vi "Configure Channels.vi"(8 "error in":errorcluster, 11 "AI Voltage DAQmx Cont CFG in":refnum<class "AI Voltage DAQmx Cont CFG.lvclass">) -> (0 "error out":errorcluster, 3 "AI Voltage DAQmx Cont CFG out":refnum<class "AI Voltage DAQmx Cont CFG.lvclass">)   [LabVIEW 2024, in "AI Voltage DAQmx Cont CFG.lvclass"]
uses:
  AI Voltage DAQmx Cont CFG.lvclass
  DAQmx BufferLastReadsDBL/DAQmx BufferLastReadsDBL.lvclass/DAQmx BufferLastReadsDBL.ctl
  DAQmx Base CFG/DAQmx Base CFG.lvclass/DAQmx Base CFG.ctl
  Configurations/CFG Base/CFG Base.lvclass/CFG Base.ctl
  a8fa0662-019b-449f-adcc-c346202d0b6d.vi
  a8fa0662-019b-449f-adcc-c346202d0b6d.vi/a4169a97-72fc-4003-a778-603cf20cafa0.vi
  <vilib>/JDP Science/JSONtext/Find Item.vi
  <vilib>/JDP Science/JSONtext/Next JSON Value.vi
  <vilib>/JDP Science/JSONtext/String Subset.vi
  <vilib>/JDP Science/JSONtext/Parsing/Advance past next JSON Value (inlined COPY).vi
  <vilib>/JDP Science/JSONtext/Parsing/Advance past whitespace.vi
  <vilib>/JDP Science/JSONtext/Parsing/Advance past String.vi
  <vilib>/JDP Science/JSONtext/Parsing/Advance past Number.vi
  <vilib>/JDP Science/JSONtext/Parsing/Advance past Line Ending.vi
  <vilib>/JDP Science/JSONtext/Parsing/Parse Full Path or Item Name.vi
  <vilib>/JDP Science/JSONtext/Parsing/Advance past Array.vi
  <vilib>/JDP Science/JSONtext/Parsing/Advance past Object.vi
  <vilib>/JDP Science/JSONtext/support/Error Cluster From Code.vi
  <vilib>/JDP Science/JSONtext/Offset/Find Item Locations by Path.vi
  <vilib>/JDP Science/JSONtext/JSON text to Variant.vi
  <vilib>/Utility/error.llb/Error Cluster From Error Code.vi
  <vilib>/DAQmx/create/channels.llb/DAQmx Create Channel (AI-Voltage-Basic).vi
  <vilib>/JDP Science/JSONtext/LVClass Serializer/JSONtext LVClass Serializer.lvclass
  DAQmx Base CFG/DAQmx Base CFG.lvclass
  DAQmx BufferLastReadsDBL/DAQmx BufferLastReadsDBL.lvclass
  Buffers/BufferLastReadingsDBL/BufferLastReadsDBL.lvclass
  Configurations/CFG Base/CFG Base.lvclass
  Configurations/CFG JSON/CFG JSON.lvclass
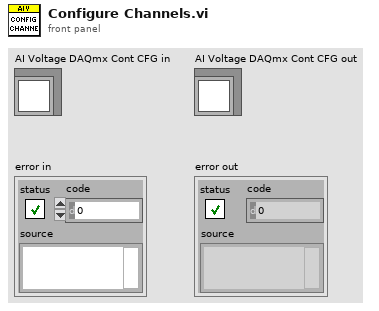
[diagram p1: front panel]
types:
  T1 = cluster{"Name":string, "Enabled":bool, "Max Value":dbl, "Min Value":dbl, "Input Terminal CFG":string, "Units":string}[]
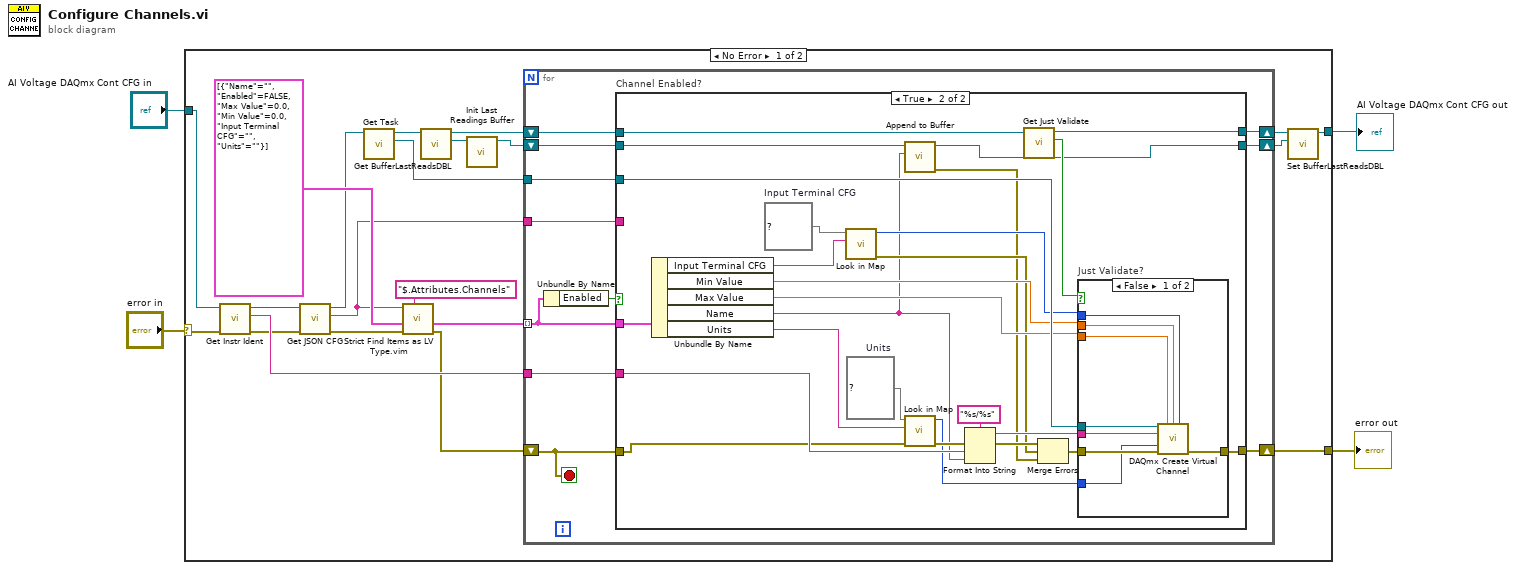
[diagram p0: block diagram]
diagram:
  n1 = case shown="No Error" "error in" {
    selector: "error in" -> [w19 w74]
    tunnel: "AI Voltage DAQmx Cont CFG in" -> [w16 w75]
    tunnel: [w20 w74] -> w1
    tunnel: [w6 w75] -> w2
    frame No Error {
      n2 = call-dynamic "Get Instr Ident.vi"("error in"=w19, "CFG JSON in"=w16) -> ("error out"=w14:errorcluster, "Instr Ident"=w21:string, "CFG JSON out"=w22:refnum<class "AI Voltage DAQmx Cont CFG.lvclass">)  [unwired: 7 in]
      n3 = call "Get JSON CFG.vi"("CFG JSON in"=w22) -> ("<JSON> CFG"=w18:string, "CFG JSON out"=w13:refnum<class "AI Voltage DAQmx Cont CFG.lvclass">)  [unwired: 9 in]
      n4 = call "Get Task.vi"("DAQmx Base CFG in"=w13) -> ("Task"=w12:refnum<k21>, "DAQmx Base CFG out"=w10:refnum<class "AI Voltage DAQmx Cont CFG.lvclass">)  [unwired: 9 in]
      n5 = call "Strict Find Items as LV Type.vim"("$Path or Item Name"="$.Attributes.Channels", "error in"=w14, "Data Type and Default Value"=T1 [{"Name"="", "Enabled"=FALSE, "Max Value"=0.0, "Min Value"=0.0, "Input Terminal CFG"="", "Units"=""}], "<JSON>"=w18) -> ("error out"=w7:errorcluster, "Data out"=w17:T1)  [unwired: 5 in, 1 out]
      n6 = call "Get BufferLastReadsDBL.vi"("DAQmx BufferLastReadsDBL in"=w10) -> ("BufferLastReadsDBL.lvclass"=w8:refnum<class "BufferLastReadsDBL.lvclass">, "DAQmx BufferLastReadsDBL out"=w9:refnum<class "AI Voltage DAQmx Cont CFG.lvclass">)  [unwired: 9 in]
      n7 = call "Init Last Readings Buffer.vi"("BufferLastReadingsDBL in"=w8) -> ("BufferLastReadingsDBL out"=w11:refnum<class "BufferLastReadsDBL.lvclass">)  [unwired: 9 in, 1 out]
      n8 = for {
        tunnel: w17 -> [w32] mode=indexing
        shift-right: [w35] -> w20
        shift-left: w7 -> [w34]
        tunnel: w21 -> [w33]
        tunnel: w18 -> [w31]
        tunnel: w12 -> [w30]
        shift-right: [w29] -> w15
        shift-left: w9 -> [w28]
        shift-right: [w25] -> w5
        shift-left: w11 -> [w26]
        stop <- w34 stop-if-true
        n9 = Unbundle By Name(w32) -> ("Enabled"=w27:bool)
        n10 = case "Channel Enabled?" shown="True" w27 {
          tunnel: [w38 w63] -> w35
          tunnel: w34 -> [w38 w45]
          tunnel: w33 -> [_ w57]
          tunnel: w32 -> [_ w64]
          tunnel: [w37 w60] -> w29
          tunnel: w31 -> [_ _]
          tunnel: w30 -> [_ w62]
          tunnel: w28 -> [w37 w61]
          tunnel: w26 -> [w36 w44]
          tunnel: [w36 w39] -> w25
          frame False {
          }
          frame True {
            w40 = map{string, i32} {"Default"=-1, "Differential"=10106, "NRSE"=10078, "Pseudodifferential"=12529, "RSE"=10083}  # Input Terminal CFG
            w41 = map{string, i32} {"From Custom Scale"=10065, "Volts"=10348}  # Units
            n11 = Unbundle By Name(w64) -> ("Input Terminal CFG"=w53:string, "Min Value"=w51:dbl, "Max Value"=w50:dbl, "Name"=w43:string, "Units"=w48:string)
            n12 = call "Look in Map.vi"("Key"=w53, "Map"=w40) -> ("error out"=w47:errorcluster, "Value"=w52:i32)  [unwired: 8 in]
            n13 = call "Append to Buffer.vi"("Channel"=w43, "BufferLastReadingsDBL in"=w44) -> ("error out"=w42:errorcluster, "BufferLastReadingsDBL out"=w39:refnum<class "BufferLastReadsDBL.lvclass">)  [unwired: 8 in]
            n14 = call "Look in Map.vi"("error in"=w45, "Key"=w48, "Map"=w41) -> ("error out"=w49:errorcluster, "Value"=w46:i32)  [unwired: 7 in]
            n15 = Format Into String(format string="%s/%s", error in=w49, w57, w43) -> (resulting string=w55:string, error out=w56:errorcluster)  [unwired: 1 in]
            n16 = call "Get Just Validate.vi"("CFG Base in"=w61) -> ("Just Validate"=w59:bool, "CFG Base out"=w60:refnum<class "AI Voltage DAQmx Cont CFG.lvclass">)  [unwired: 9 in]
            n17 = Merge Errors(w56, w47, w42) -> (w54:errorcluster)
            n18 = case "Just Validate?" shown="False" w59 {
              tunnel: w54 -> [w72 w73]
              tunnel: w55 -> [w69 _]
              tunnel: w62 -> [w71 _]
              tunnel: [w70 w73] -> w63
              tunnel: w52 -> [w65 _]
              tunnel: w51 -> [w68 _]
              tunnel: w50 -> [w67 _]
              tunnel: w46 -> [w66 _]
              frame False {
                n19 = call-poly <vilib>:"DAQmx Create Virtual Channel.vi"("task in"=w71, "maximum value"=w67, "minimum value"=w68, "input terminal configuration"=w65, "physical channels"=w69, "units"=w66, "error in"=w72) -> ("error out"=w70:errorcluster)  [unwired: 7 in, 1 out]
              }
              frame True {
              }
            }
          }
        }
      }
      n20 = call "Set BufferLastReadsDBL.vi"("BufferLastReadsDBL.lvclass"=w5, "DAQmx BufferLastReadsDBL in"=w15) -> ("DAQmx BufferLastReadsDBL out"=w6:refnum<class "AI Voltage DAQmx Cont CFG.lvclass">)  [unwired: 9 in]
    }
    frame Error {
    }
  }
  "error out" <- w1
  "AI Voltage DAQmx Cont CFG out" <- w2
